vi "Operaciones diferentes casos.vi"() -> ()   [LabVIEW 2020]
panel:
  in  "Enum":enum16{"SUMA", "RESTA", "MULT", "DIV"}(ring)
  out "RESUL":dbl
  in  "NUM 2":dbl
  in  "NUM1":dbl
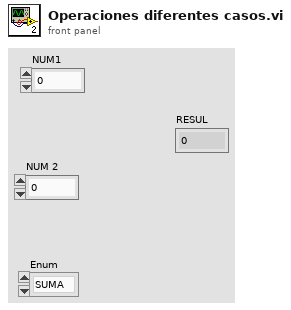
[diagram p1: front panel]
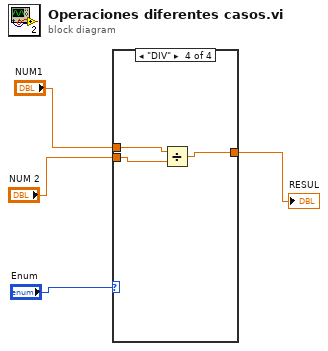
[diagram p0: block diagram]
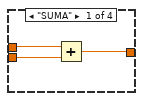
[diagram p2: hidden frame]
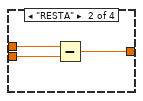
[diagram p3: hidden frame]
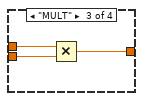
[diagram p4: hidden frame]
diagram:
  n1 = case shown="\"DIV\"" "Enum" {
    tunnel: "NUM1" -> [w7 w10 w13 w16]
    tunnel: "NUM 2" -> [w6 w9 w12 w15]
    tunnel: [w5 w8 w11 w14] -> w1
    frame "SUMA" {
      n2 = Add(x=w7, y=w6) -> (x+y=w5:dbl)
    }
    frame "RESTA" {
      n3 = Subtract(x=w10, y=w9) -> (x-y=w8:dbl)
    }
    frame "MULT" {
      n4 = Multiply(x=w13, y=w12) -> (x*y=w11:dbl)
    }
    frame "DIV" {
      n5 = Divide(x=w16, y=w15) -> (x/y=w14:dbl)
    }
  }
  "RESUL" <- w1
